vi "Post-Build Action Launcher.vi"(5 "Files Generated by Build":path[](array[path]), 6 "Top Level/Always Included VIs":path[](array[path]), 7 "Destination Path":path, 8 "error in (no error)":errorcluster, 9 "Target Name":string, 10 "Build Specification Name":string, 11 "Project Path":path) -> (0 "error out":errorcluster)   [LabVIEW 2019, in "Package Builder.lvlib"]
uses:
  Package Builder.lvlib
  TypeDefs/Post-Build Action Launcher States.ctl
  TypeDefs/Post-Build Action Launcher IDC.ctl
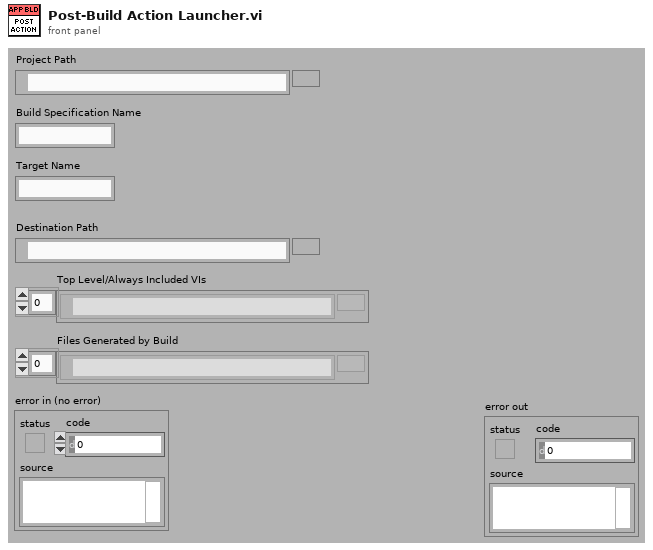
[diagram p1: front panel]
types:
  T1 = typedef "Package Builder.lvlib/Post-Build Action Launcher States.ctl" = enum16{"Initialize", "Shutdown", "Build Package", "Build All Specifications", "Wait for Confirimation", "Error"}
  T2 = typedef "Package Builder.lvlib/Post-Build Action Launcher IDC.ctl" = cluster{"Project Path":path, "Build Specifications":string[], "Build Specification Name":string, "Package Build Specification":string, "Target Name":string, "Destination Path":path, "Top Level/Always Included VIs":path[], "Files Generated by Build":path[]}
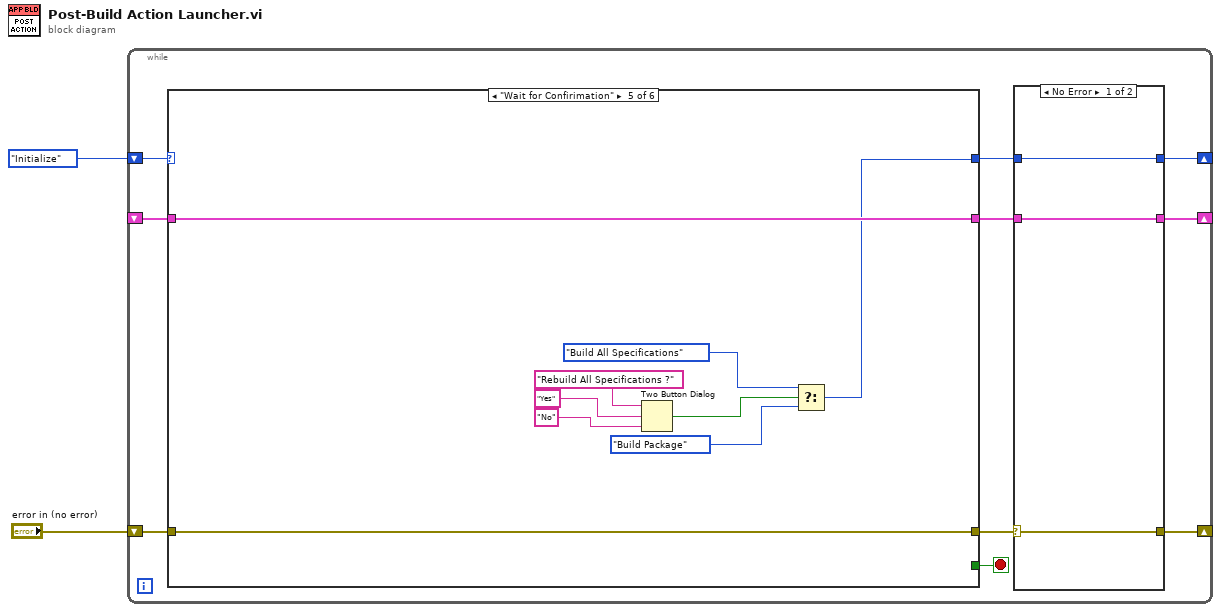
[diagram p0: block diagram]
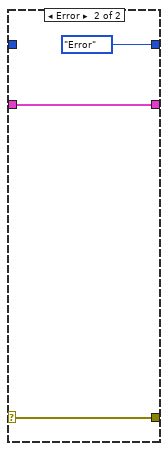
[diagram p2: hidden frame]
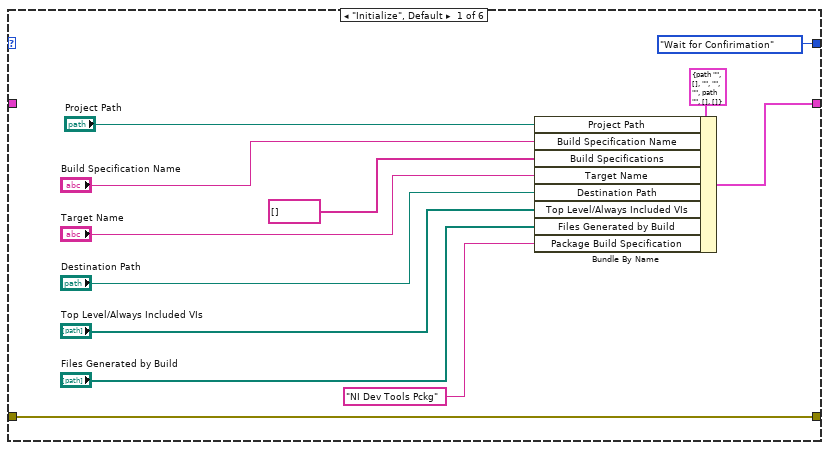
[diagram p3: hidden frame]
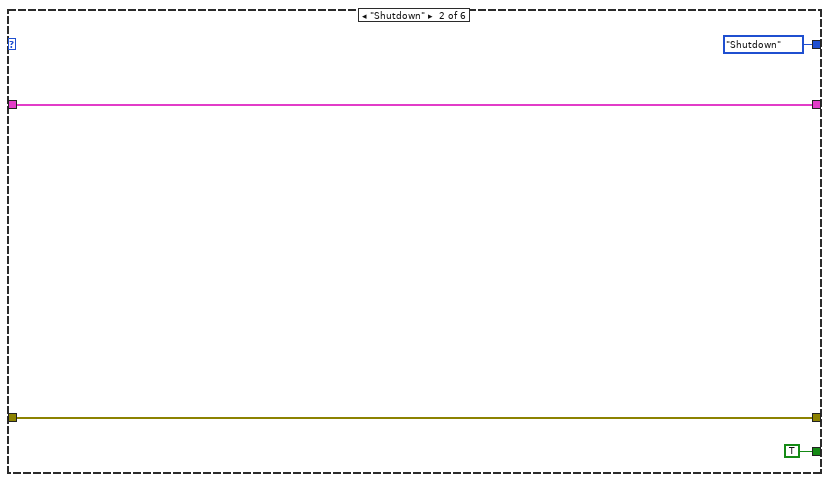
[diagram p4: hidden frame]
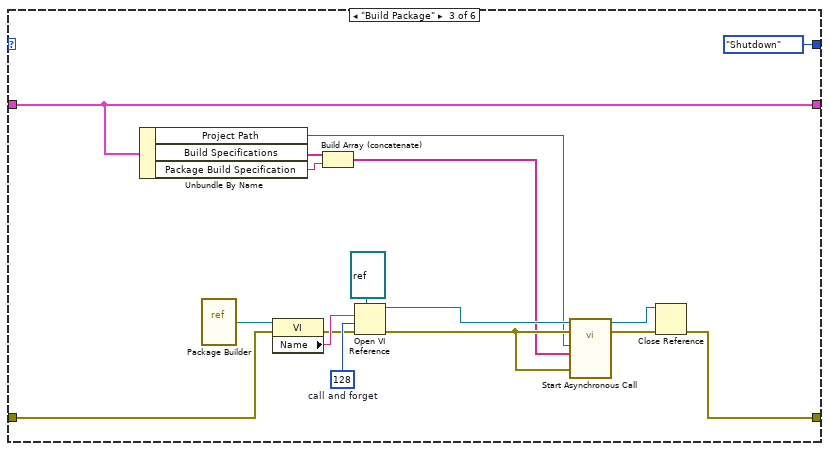
[diagram p5: hidden frame]
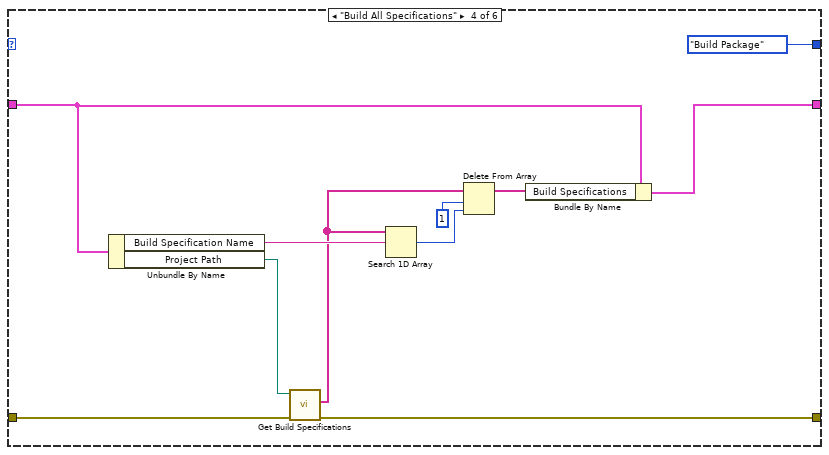
[diagram p6: hidden frame]
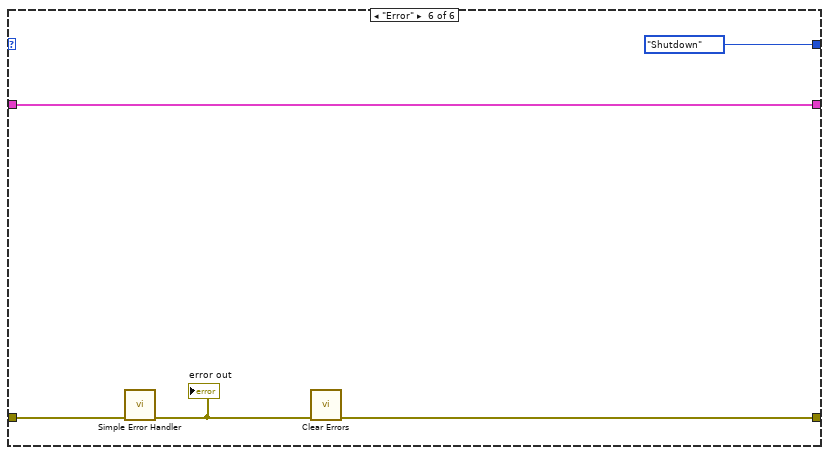
[diagram p7: hidden frame]
diagram:
  n1 = while {
    shift-right: [w4] -> _
    shift-left: _ -> [w11]
    shift-right: [w8] -> _
    shift-left: "error in (no error)" -> [w10]
    shift-right: [w7] -> _
    shift-left: Post-Build_Action_Launcher_States."Initialize" -> [w12]
    stop <- w3 stop-if-true
    n2 = case shown="\"Wait for Confirimation\"" w12 {
      tunnel: [w25 w33 w39 w58 w70 w74] -> w5
      tunnel: w11 -> [_ w33 w39 w59 w70 w74]
      tunnel: w10 -> [w24 w32 w41 w61 w71 w76]
      tunnel: [w24 w32 w40 w57 w71 w73] -> w9
      tunnel: [Post-Build_Action_Launcher_States."Wait for Confirimation" Post-Build_Action_Launcher_States."Shutdown" Post-Build_Action_Launcher_States."Shutdown" Post-Build_Action_Launcher_States."Build Package" w65 Post-Build_Action_Launcher_States."Shutdown"] -> w6
      tunnel: [_ TRUE _ _ _ _] -> w3
      frame "Initialize", Default {
        n3 = Bundle By Name(cluster=T2 {"Project Path"=path "", "Build Specifications"=[], "Build Specification Name"="", "Package Build Specification"="", "Target Name"="", "Destination Path"=path "", "Top Level/Always Included VIs"=[], "Files Generated by Build"=[]} ("Internal Data Cluster"), "Project Path"="Project Path", "Build Specification Name"="Build Specification Name", "Build Specifications"=string[] [], "Target Name"="Target Name", "Destination Path"="Destination Path", "Top Level/Always Included VIs"="Top Level/Always Included VIs", "Files Generated by Build"="Files Generated by Build", "Package Build Specification"="NI Dev Tools Pckg") -> (w25:T2)
      }
      frame "Shutdown" {
      }
      frame "Build Package" {
        w50 = 128  # call and forget
        n4 = Unbundle By Name(w39) -> ("Project Path"=w36:path, "Build Specifications"=w38:string[], "Package Build Specification"=w37:string)
        n5 = vi-ref "Package Builder.vi"() -> (w49:refnum<vi>)
        n6 = property class="VI"(reference=w49, error in=w41) -> (error out=w47:errorcluster, "Name"=w48:string)  [unwired: 1 out]
        n7 = Build Array (concatenate)(w38, w37) -> (w35:string[])
        n8 = Open VI Reference(type specifier VI Refnum (for type only)=refnum<vi> refnum, vi path=w48, options=w50, error in (no error)=w47) -> (vi reference=w44:refnum<vi>, error out=w46:errorcluster)  [unwired: 2 in]
        n9 = call-by-ref "Start Asynchronous Call"(reference=w44, error in=w46, "error in"=w46, "Build Specifications"=w35, "Project Path"=w36) -> (reference out=w43:refnum<vi>, error out=w45:errorcluster)  [unwired: 8 in, 1 out]
        n10 = Close Reference(reference=w43, error in (no error)=w45) -> (error out=w40:errorcluster)
      }
      frame "Build All Specifications" {
        n11 = Unbundle By Name(w59) -> ("Build Specification Name"=w56:string, "Project Path"=w60:path)
        n12 = call "Get Build Specifications.vi"("error in (no error)"=w61, "Project Path in"=w60) -> ("error out"=w57:errorcluster, "Build Specification Names"=w54:string[])  [unwired: 7 in, 1 out]
        n13 = Search 1D Array(1D array=w54, element=w56) -> (index of element=w55:i32)  [unwired: 1 in]
        n14 = Delete From Array(array=w54, length=1, index=w55) -> (array with subset deleted=w52:string[])  [unwired: 1 out]
        n15 = Bundle By Name(cluster=w59, "Build Specifications"=w52) -> (w58:T2)
      }
      frame "Wait for Confirimation" {
        n16 = Two Button Dialog(message="Rebuild All Specifications ?", 1:"No" ("F button name (\"Cancel\")"), 2:"Yes" ("T button name (\"OK\")")) -> (T button?=w67:bool)
        n17 = Select(t=Post-Build_Action_Launcher_States."Build All Specifications", s=w67, f=Post-Build_Action_Launcher_States."Build Package") -> (s? t:f=w65:T1)
      }
      frame "Error" {
        n18 = call <vilib>:"Simple Error Handler.vi"("error in (no error)"=w76) -> ("error out"=w72:errorcluster)  [unwired: 4 in, 4 out]
        "error out" <- w72
        n19 = call <vilib>:"Clear Errors.vi"("error in (no error)"=w72) -> ("error out"=w73:errorcluster)  [unwired: 5 in, 1 out]
      }
    }
    n20 = case shown="No Error" w9 {
      selector: w9 -> [w15 w16]
      tunnel: [w15 w16] -> w8
      tunnel: [w14 Post-Build_Action_Launcher_States."Error"] -> w7
      tunnel: w6 -> [w14 _]
      tunnel: w5 -> [w13 w17]
      tunnel: [w13 w17] -> w4
      frame No Error {
      }
      frame Error {
      }
    }
  }
